vi "2014 Target Detection[1].vi"() -> (2 "Target Info":T5(array[cluster]))   [LabVIEW 2013]
uses:
  <vilib>/Rock Robotics/WPI/Camera/WPI_CameraSettings Read MJPG.ctl
  <vilib>/Rock Robotics/WPI/Camera/WPI_CameraImageSize.ctl
  2014 Target Detection/TargetType.ctl
panel:
  in  "Range":cluster{"Lower value":sgl, "Upper value":sgl}={"Lower value"=150.0, "Upper value"=255.0} {"Lower value" scale=0.0..255.0; "Upper value" scale=0.0..255.0}
  in  "Instructions:":string="Images:\nUse the tab immediately below to choose the image source. Update the camera settings or the image directory so that you have images or video to test with.\n\nCalibration:\nYou can update Color Component ranges directly, or by clicking and drawing a line on the colored strip in the Image control. The Std Dev multipliers and where the strip is drawn determine the calibration values.\n\nUse Debugging tab to view the result of the color range threshold .\n\nArea Size LImit is used to ignore objects too small or far away to care about.\n\nThe Details tab contains score details for each target and subObject.\n\nCamera Type is used to select lens angles for distance calculation.\n\nVertical strips with no adjacent horizontal strip are identified as \"not hot\" and marked in blue.\nThe numeric scores indicate represent aspect ratio and rectangularity.\n\nWhen both strips are near enough, the pair is identified as \"hot\" and marked in green. Scores\nindicate the left, right, ratio of widths, and vertical positioning.\n\nAny score that falls below cutoff is drawn in red and bounding box is drawn in red."
  in  "Std Devs":cluster{"Hue":dbl, "Sat":dbl, "Val":dbl}={"Hue"=4.0, "Sat"=6.0, "Val"=4.0}
  in  "Area Size Limit %":dbl=0.06 format="%#_13g"
  in  "Camera Type":enum16{"206", "1011", "1013"}(ring)=enum."1013"
  out "loop time ms":u32
  in  "Score Cutoff":dbl(slide)=54.248366013071895 scale=0.0..100.0
  out "Error":bool
  in  "Image Source":enum32{"Files", "Camera"}(tab)
  in  "List of image files":i32(listbox)
  in  "Image Directory":path=path "2014 Pseudo-Target/2014 Pseudo-Target Active"
  in  "Camera Settings":T1={"fps"=15, "compression"=5, "Image Size"=enum."320x240"}
  in  "Camera IP":string="10.00.00.11"
  in  "Tabbed Info":enum32{"Debugging", "Details"}(tab)
  out "Mask":T3(plugin-control)
  out "Image":T3(plugin-control)
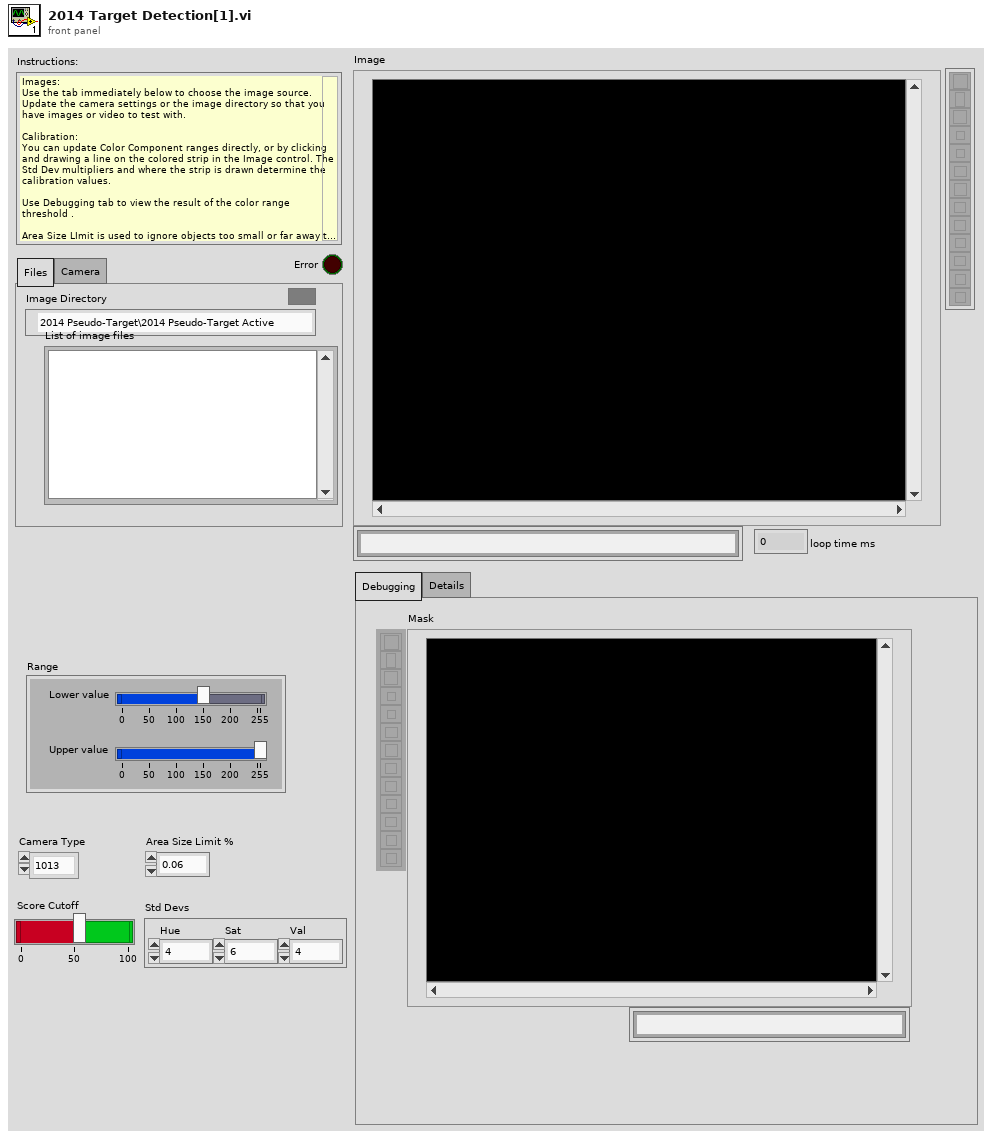
[diagram p1: front panel]
types:
  T1 = typedef "WPI_CameraSettings Read MJPG.ctl" = cluster{"fps":i32, "compression":i32, "Image Size":T2}
  T2 = typedef "WPI_CameraImageSize.ctl" = enum16{"640x480", "320x240", "160x120"}
  T3 = typedef "IMAQ Image.ctl" = refnum<image>
  T4 = typedef "TargetType.ctl" = enum16{"Not Hot", "Hot"}
  T5 = cluster{"Scores":cluster{"Total":dbl, "Left":dbl, "Right":dbl, "Ratio":dbl, "Vertical":dbl, "index":i32, "State":T4}, "Verticals":cluster{"Horizontal?":bool, "Aspect Score":dbl, "Rect Score":dbl, cluster{"Left":dbl, "Top":dbl, "Right":dbl, "Bottom":dbl}, "Equiv H":dbl, "Equiv V":dbl}, "Horizontals":cluster{"Horizontal?":bool, "Aspect Score":dbl, "Rect Score":dbl, cluster{"Left":dbl, "Top":dbl, "Right":dbl, "Bottom":dbl}, "Equiv H":dbl, "Equiv V":dbl}, "Distance ft":dbl, "Center":cluster{"X":dbl, "Y":dbl}}[]
  T6 = typedef "Image Type" = u32
  T7 = typedef "WPI_CameraDevRef.ctl" = cluster{"Camera Address":string, "CameraStatus":errorcluster, "Acquire Image Notifier":refnum<notifier>}
  T8 = cluster{"Horizontal":bool, "Aspect Score":dbl, "Rect Score":dbl, cluster{"Left":dbl, "Top":dbl, "Right":dbl, "Bottom":dbl}, "Equiv H":dbl, "Equiv V":dbl}[]
  T9 = cluster{cluster{dbl, dbl}, cluster{dbl, dbl}, cluster{dbl, dbl}}
  T10 = cluster{"Scores":cluster{"Total":dbl, "Left":dbl, "Right":dbl, "Ratio":dbl, "Vertical":dbl, "index":i32, "State":T4}, "Verticals":cluster{"Horizontal?":bool, "Aspect Score":dbl, "Rect Score":dbl, cluster{"Left":dbl, "Top":dbl, "Right":dbl, "Bottom":dbl}, "Equiv H":dbl, "Equiv V":dbl}, "Horizontals":cluster{"Horizontal?":bool, "Aspect Score":dbl, "Rect Score":dbl, cluster{"Left":dbl, "Top":dbl, "Right":dbl, "Bottom":dbl}, "Equiv H":dbl, "Equiv V":dbl}, "Validated":bool}[]
  T11 = cluster{"Scores":cluster{"Total":dbl, "Left":dbl, "Right":dbl, "Ratio":dbl, "Vertical":dbl, "index":i32, "State":T4}, "Verticals":cluster{"Horizontal?":bool, "Aspect Score":dbl, "Rect Score":dbl, cluster{"Left":dbl, "Top":dbl, "Right":dbl, "Bottom":dbl}, "Equiv H":dbl, "Equiv V":dbl}, "Horizontals":cluster{"Horizontal?":bool, "Aspect Score":dbl, "Rect Score":dbl, cluster{"Left":dbl, "Top":dbl, "Right":dbl, "Bottom":dbl}, "Equiv H":dbl, "Equiv V":dbl}, "Distance (ft)":dbl, "Target Center (-1 to 1)":cluster{"X":dbl, "Y":dbl}}[]
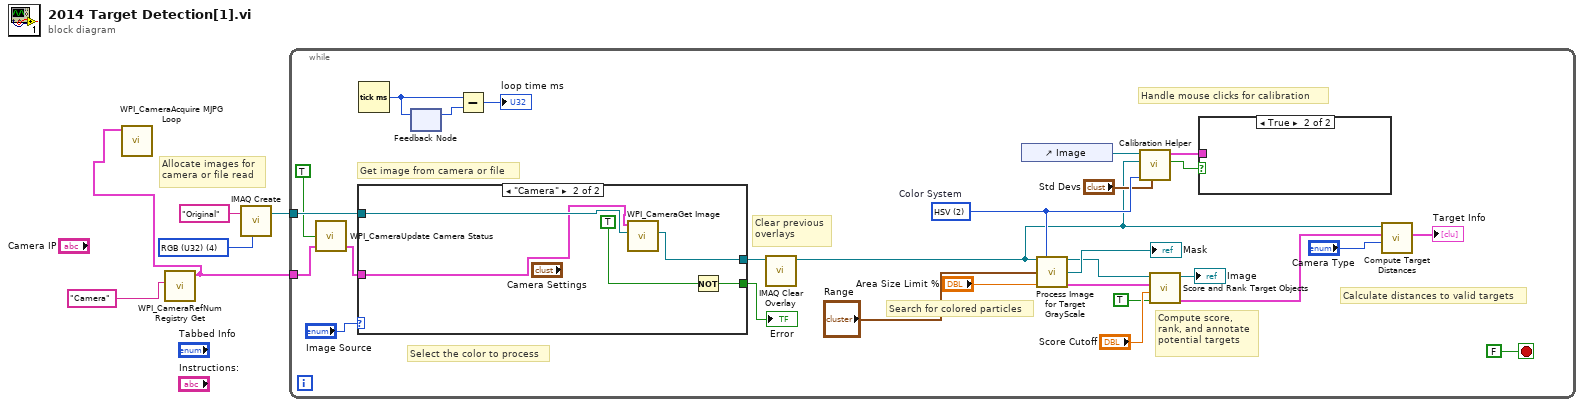
[diagram p0: block diagram]
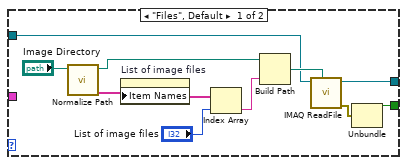
[diagram p3: hidden frame]
diagram:
  w5 = T6 4 items=["Grayscale (U8)", "Grayscale (I16)", "Grayscale (SGL)", "Complex (CSG)", "RGB (U32)", "HSL (U32)", "RGB (U64)", "Grayscale (U16)"] ("Image Type")
  # "Allocate images for\ncamera or file read"
  n1 = call <vilib>:"WPI_CameraRefNum Registry Get.vi"("refnum name"="Camera") -> ("CameraDevRef"=w1:T7)  [unwired: 9 in, 1 out]
  n2 = call <vilib>:"WPI_CameraAcquire MJPG Loop.vi"("CameraDevRef"=w1) -> ()  [unwired: 11 in]
  n3 = call "IMAQ Create"("Image Name"="Original", "Image Type"=w5) -> ("New Image"=w3:T3)  [unwired: 3 in, 1 out]
  n4 = while {
    tunnel: w3 -> [w30]
    tunnel: w1 -> [w7]
    stop <- FALSE stop-if-true
    w15 = u16 2 items=["RGB", "HSL", "HSV", "HSI"]  # Color System
    # "Clear previous\noverlays"
    # "Calculate distances to valid targets"
    # "Search for colored particles"
    # "Handle mouse clicks for calibration"
    # "Compute score,\nrank, and annotate\npotential targets"
    # "Select the color to process"
    # "Get image from camera or file"
    n5 = call <vilib>:"WPI_CameraUpdate Camera Status.vi"("CameraDevRef In"=w7, "Enable Vision"=TRUE) -> ("CameraDevRef Out"=w6:T7)  [unwired: 3 in]
    n6 = case shown="\"Camera\"" "Image Source" {
      tunnel: [w40 w46] -> w33
      tunnel: w30 -> [w39 w47]
      tunnel: [w37 w48] -> w29
      tunnel: w6 -> [_ w44]
      frame "Files", Default {
        n7 = call "Normalize Path.vi"("Image Directory"="Image Directory") -> ("Filenames"=w35:string[], "Path"=w34:path)  [unwired: 9 in]
        n8 = property on="List of image files" class="LstBox (strict)"("Item Names"=w35) -> ()  [unwired: 2 in, 2 out]
        n9 = Index Array(array=w35, index="List of image files") -> (element=w42:string)
        n10 = Build Path(base path=w34, name or relative path=w42) -> (appended path=w41:path)
        n11 = call "IMAQ ReadFile"("File Path"=w41, "Image"=w39) -> ("error out"=w38:errorcluster, "Image Out"=w40:T3)  [unwired: 5 in, 3 out]
        n12 = Unbundle(w38) -> ("status"=w37:bool)  [unwired: 2 out]
      }
      frame "Camera" {
        n13 = call <vilib>:"WPI_CameraGet Image.vi"("Image"=w47, "CameraDevRef"=w44) -> ("Image Out"=w46:T3)  [unwired: 7 in, 2 out]
        n14 = Not(x=TRUE ("Enable")) -> (.not. x?=w48:bool)
      }
    }
    "Error" <- w29
    n15 = Tick Count (ms)() -> (millisecond timer value=w28:u32)
    n16 = feedback #1() -> (w27:u32)  [unwired: 1 in]
    n17 = feedback-in #1(w28) -> ()
    n18 = Subtract(x=w28, y=w27) -> (x-y=→"loop time ms":u32)
    n19 = call "IMAQ Clear Overlay"("Image"=w33) -> ("Image Out"=w11:T3)  [unwired: 9 in, 1 out]
    n20 = control-ref of="Image"() -> (w16:refnum<vi>)
    n21 = call "Process Image for Target GrayScale.vi"("Src Image"=w11, "Color Mode"=w15, "Range"="Range", "Area Cutoff %"="Area Size Limit %") -> ("Src Image Out"=w23:T3, "Threshold"=→"Mask":T3, "Particles"=w20:T8)  [unwired: 9 in]
    n22 = call "Calibration Helper.vi"("Std Devs"="Std Devs", "Color Mode"=w15, "Image"=w11, "Image Ctl Refnum"=w16) -> ("Changed"=w12:bool, "output color"=w13:T9)  [unwired: 6 in]
    n23 = call "Score and Rank Target Objects.vi"("Annotate"=TRUE, "Score Limit"="Score Cutoff", "Particles"=w20, "Image in"=w23) -> ("Target Info"=w19:T10, "Annotated Image"=→"Image":T3)  [unwired: 6 in]
    n24 = case shown="True" w12 {
      tunnel: w13 -> [_ _]
      frame False {
      }
      frame True {
      }
    }
    n25 = call "Compute Target Distances.vi"("Camera Type"="Camera Type", "Target Info"=w19, "Image in"=w11) -> ("Target Info"=→"Target Info":T11)  [unwired: 6 in, 2 out]
  }
